vi "Create.vi"(8 "Error In":errorcluster, 11 "Object":refnum<class "CS++Base.lvclass">) -> (0 "Error Out":errorcluster, 2 "Created new?":bool, 3 "Object Reference":refnum<class "CS++Reference.lvclass">)   [LabVIEW 2015, in "CS++BaseClasses.lvlib" / "CS++Reference.lvclass"]
doc: "Create an object reference.\n\nInsert object into single element sized queue and retrun the reference object, that can be cloned without cloning the contained object."
uses:
  CS++Reference.lvclass
  Base/CS++Base.lvclass
  Base/CS++Base.lvclass/CS++Base.ctl
  CS++Reference.lvclass/CS++Reference.ctl
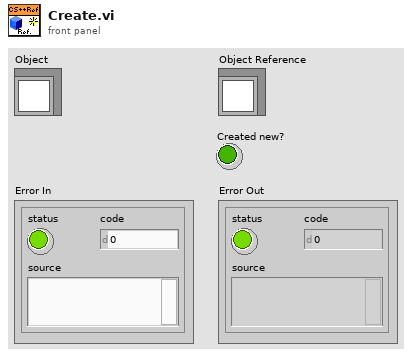
[diagram p1: front panel]
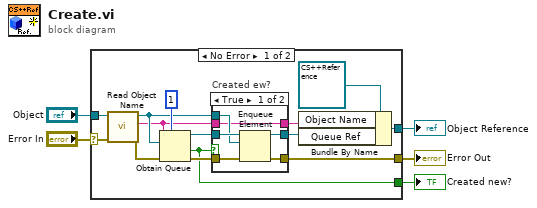
[diagram p0: block diagram]
diagram:
  n1 = case shown="No Error" "Error In" {
    selector: "Error In" -> [w6 w29]
    tunnel: "Object" -> [w19 _]
    tunnel: [w12 w29] -> w4
    tunnel: [w11 _] -> w3
    tunnel: [w7 _] -> w1
    frame No Error {
      n2 = call "Read Object Name.vi"("error in (no error)"=w6, "Base in"=w19) -> ("error out"=w18:errorcluster, "Object Name"=w13:string, "Base out"=w14:refnum<class "CS++Base.lvclass">)  [unwired: 7 in]
      n3 = Obtain Queue(max queue size (-1, unlimited)=1, name (unnamed)=w13, element data type=w14, error in (no error)=w18) -> (queue out=w16:refnum<queue>, created new?=w11:bool, error out=w15:errorcluster)  [unwired: 1 in]
      n4 = case "Created ew?" shown="True" w11 {
        tunnel: w16 -> [w25 w27]
        tunnel: w15 -> [w24 w28]
        tunnel: w14 -> [w23 _]
        tunnel: w13 -> [w20 w26]
        tunnel: [w21 w27] -> w8
        tunnel: [w22 w28] -> w12
        tunnel: [w20 w26] -> w9
        frame True {
          n5 = Enqueue Element(queue=w25, element=w23, error in (no error)=w24) -> (queue out=w21:refnum<queue>, error out=w22:errorcluster)  [unwired: 1 in, 1 out]
        }
        frame False {
        }
      }
      n6 = Bundle By Name(cluster=refnum<class "CS++Reference.lvclass"> refnum ("Object Reference"), "Object Name"=w9, "Queue Ref"=w8) -> (w7:refnum<class "CS++Reference.lvclass">)
    }
    frame Error {
    }
  }
  "Error Out" <- w4
  "Created new?" <- w3
  "Object Reference" <- w1
